vi "Uniform Inverse CDF.vi"(9 "xmax":dbl=1.0, 10 "xmin":dbl, 11 "cdf(x)":dbl=1.0) -> (0 "error":i32, 3 "x":dbl=1.0)   [LabVIEW 2017, in "NI_Gmath.lvlib"]
doc: "Computes the continuous inverse cumulative distribution function (CDF) of the various distributions. You must manually select the polymorphic instance to use."
uses:
  NI_Gmath.lvlib
  st_error_code.ctl
panel:
  # "Uniform Inverse CDF"
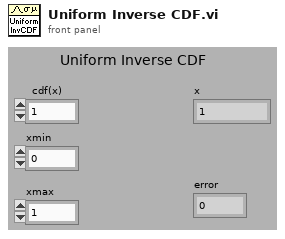
[diagram p1: front panel]
types:
  T1 = typedef "NI_Gmath.lvlib/st_error_code.ctl" = i32
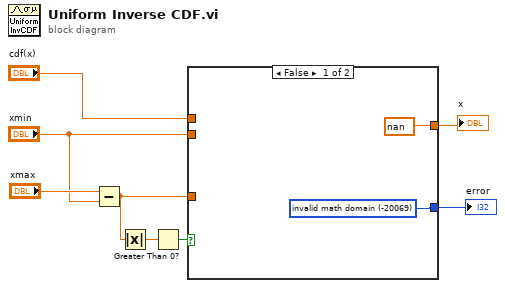
[diagram p0: block diagram]
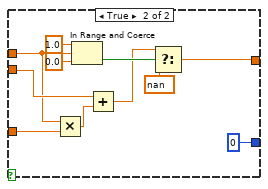
[diagram p2: hidden frame]
diagram:
  n1 = Subtract(x="xmax", y="xmin") -> (x-y=w4:dbl)
  n2 = Absolute Value(x=w4) -> (abs(x)=w5:dbl)
  n3 = Greater Than 0?(x=w5) -> (x > 0?=w3:bool)
  n4 = case shown="False" w3 {
    tunnel: "cdf(x)" -> [_ w15]
    tunnel: "xmin" -> [_ w16]
    tunnel: w4 -> [_ w14]
    tunnel: [nan w11] -> w2
    tunnel: [w9 0] -> w1
    frame False {
      w9 = T1 -20069 items=["invalid math domain"=-20069, "Fourier interpolation size m >= n"=-20070, "empty array"=-20003] ("stat interp error code")
    }
    frame True {
      n5 = Multiply(x=w15, y=w14) -> (x*y=w13:dbl)
      n6 = In Range and Coerce(upper limit=1.0, x=w15, lower limit=0.0) -> (In Range?=w18:bool)  [unwired: 1 out]
      n7 = Add(x=w16, y=w13) -> (x+y=w12:dbl)
      n8 = Select(t=w12, s=w18, f=nan) -> (s? t:f=w11:dbl)
    }
  }
  "x" <- w2
  "error" <- w1
